vi "PixyHexDecode.vi"(0 "Object":string) -> (4 "Color Code":dbl, 6 "X":dbl, 8 "Y":dbl, 10 "Width":dbl, 15 "Height":dbl)   [LabVIEW 2016]
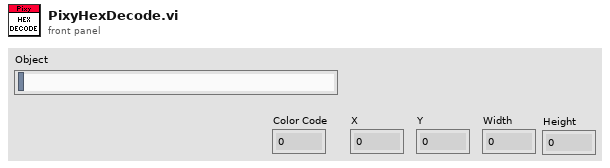
[diagram p1: front panel]
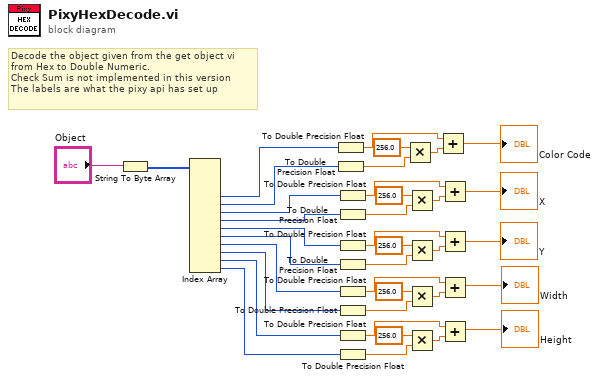
[diagram p0: block diagram]
diagram:
  # "Decode the object given from the get object vi\nfrom Hex to Double Numeric.\nCheck Sum is not implemented in this version\nThe labels are what the pixy api has set up"
  n1 = String To Byte Array(string="Object") -> (unsigned byte array=w36:u8[])
  n2 = Index Array(array=w36) -> (element #3=w10:u8, element #4=w9:u8, element #5=w8:u8, element #6=w7:u8, element #7=w6:u8, element #8=w5:u8, element #9=w4:u8, element #10=w3:u8, element #11=w2:u8, element #12=w1:u8)  [unwired: 12 in, 2 out]
  n3 = To Double Precision Float(number=w10) -> (double precision float=w32:dbl)
  n4 = To Double Precision Float(number=w9) -> (double precision float=w34:dbl)
  n5 = To Double Precision Float(number=w8) -> (double precision float=w28:dbl)
  n6 = To Double Precision Float(number=w7) -> (double precision float=w30:dbl)
  n7 = To Double Precision Float(number=w6) -> (double precision float=w24:dbl)
  n8 = To Double Precision Float(number=w5) -> (double precision float=w26:dbl)
  n9 = To Double Precision Float(number=w4) -> (double precision float=w20:dbl)
  n10 = To Double Precision Float(number=w3) -> (double precision float=w22:dbl)
  n11 = To Double Precision Float(number=w2) -> (double precision float=w16:dbl)
  n12 = To Double Precision Float(number=w1) -> (double precision float=w18:dbl)
  n13 = Multiply(x=256.0, y=w34) -> (x*y=w33:dbl)
  n14 = Multiply(x=256.0, y=w30) -> (x*y=w29:dbl)
  n15 = Multiply(x=256.0, y=w26) -> (x*y=w25:dbl)
  n16 = Multiply(x=256.0, y=w22) -> (x*y=w21:dbl)
  n17 = Multiply(x=256.0, y=w18) -> (x*y=w17:dbl)
  n18 = Add(x=w32, y=w33) -> (x+y=→"Color Code":dbl)
  n19 = Add(x=w28, y=w29) -> (x+y=→"X":dbl)
  n20 = Add(x=w24, y=w25) -> (x+y=→"Y":dbl)
  n21 = Add(x=w20, y=w21) -> (x+y=→"Width":dbl)
  n22 = Add(x=w16, y=w17) -> (x+y=→"Height":dbl)
